vi "Create Group Logger.vi"(7 "Timestamp":string, 8 "error in (no error)":errorcluster, 10 "Group":refnum<class "Group.lvclass">, 11 "Historian Logger in":refnum<class "Historian Logger.lvclass">) -> (0 "error out":errorcluster, 3 "Historian Logger out":refnum<class "Historian Logger.lvclass">)   [LabVIEW 2020, in "VolatusHistorian.lvlib" / "Historian Logger.lvclass"]
uses:
  Historian Logger.lvclass
  C:/dev/lv20CE/relink/lv-volatus/Volatus/Module/Module.lvclass
  lv-vecto/Vecto/Group/Group.lvclass
  Group Buffer DBL/Group Buffer DBL.lvclass
  Volatus/Module/Module.lvclass/Module.ctl
  lv-vecto/Vecto/Group/Group.lvclass/Group.ctl
  lv-vecto/Vecto/Group Config/Group Config.lvclass/Group Config.ctl
  lv-vecto/Vecto/Group DBL/Group DBL.lvclass
  Group Info.ctl
  Volatus/MessageQ/MessageQ.lvclass
  VolatusData/Logger State.ctl
  VolatusConfig/VolatusConfigElement/VolatusConfigElement.lvclass
  Historian Logger.lvclass/Historian Logger.ctl
  VolatusData/Data Logger DBL Module/Data Logger DBL Module.lvclass
  Volatus/Module/Module.lvclass
  VolatusData/VolatusData.lvlib
  C:/dev/lv20CE/relink/lv-volatus/VolatusHistorian/Historian Logger/Historian Logger.lvclass
  C:/dev/lv20CE/relink/lv-volatus/VolatusData/Data Logger DBL Module/Data Logger DBL Module.lvclass
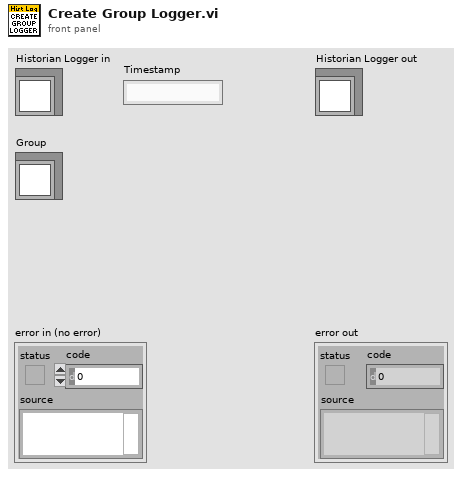
[diagram p1: front panel]
types:
  T1 = typedef "VectoConfig.lvlib/Group Data Type.ctl" = enum16{"Double", "String", "Bool"}
  T2 = typedef "VolatusData.lvlib/Prepare Log.ctl" = cluster{"Folder":path, "Series":string}
  T3 = typedef "VolatusHistorian.lvlib/Historian Logger.lvclass/Group Info.ctl" = cluster{"Buffer":refnum<class "Group Buffer DBL.lvclass">, "Logger":refnum<class "MessageQ.lvclass">, "Group":refnum<class "Group.lvclass">, "Last Timestamp":dbl, "State":T4}
  T4 = typedef "VolatusData.lvlib/Logger State.ctl" = enum16{"Unknown", "Idle", "Preparing", "Ready", "Logging", "Stopping"}
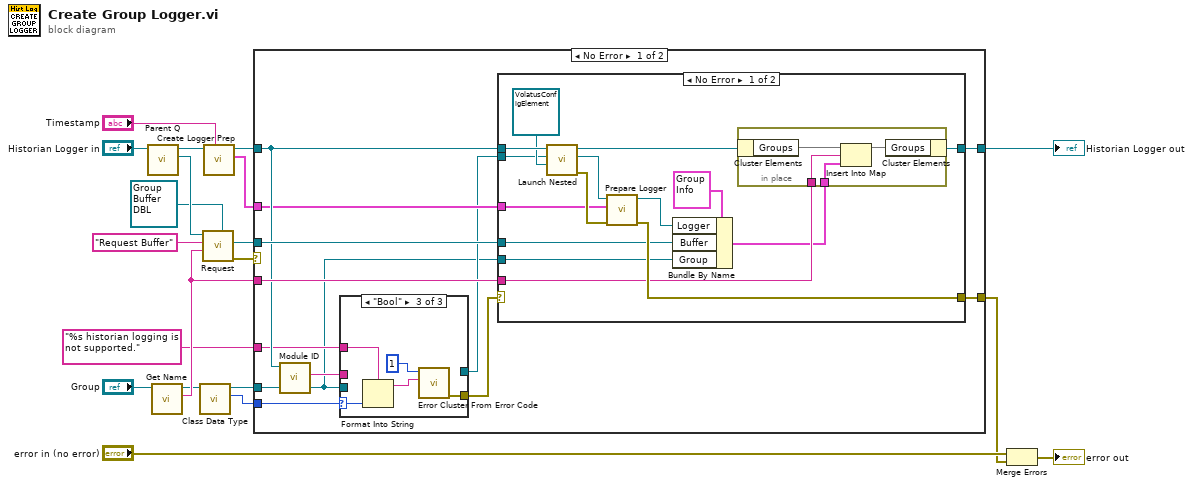
[diagram p0: block diagram]
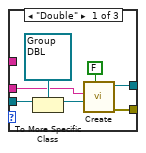
[diagram p2: hidden frame]
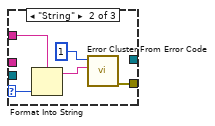
[diagram p3: hidden frame]
diagram:
  n1 = call "Parent Q.vi"("Module in"="Historian Logger in") -> ("Parent Q"=w16:refnum<class "MessageQ.lvclass">, "Module out"=w8:refnum<class "Historian Logger.lvclass">)  [unwired: 9 in]
  n2 = call "Get Name.vi"("Group in"="Group") -> ("Name"=w12:string, "Group out"=w5:refnum<class "Group.lvclass">)  [unwired: 8 in, 1 out]
  n3 = call "Class Data Type.vi"("Group in"=w5) -> ("Class Data Type"=w4:T1, "Group out"=w3:refnum<class "Group.lvclass">)  [unwired: 8 in, 1 out]
  n4 = call "Request.vi"("Response Type (None)"=refnum<class "Group Buffer DBL.lvclass"> refnum ("VolatusHistorian.lvlib:Group Buffer DBL.lvclass"), "Data"=w12, "ID"="Request Buffer", "MessageQ in"=w16) -> ("error out"=w14:errorcluster, "Response"=w13:refnum<class "Group Buffer DBL.lvclass">)  [unwired: 5 in, 1 out]
  n5 = call "Create Logger Prep.vi"("Timestamp"="Timestamp", "Historian Logger in"=w8) -> ("Logger Info"=w6:T2, "Historian Logger out"=w7:refnum<class "Historian Logger.lvclass">)  [unwired: 7 in, 1 out]
  n6 = case shown="No Error" w14 {
    selector: w14 -> [_ w72]
    tunnel: w13 -> [w29 _]
    tunnel: w7 -> [w28 w71]
    tunnel: w12 -> [w30 _]
    tunnel: [w27 w71] -> w11
    tunnel: [w31 w72] -> w9
    tunnel: w6 -> [w26 _]
    tunnel: w4 -> [w25 _]
    tunnel: w3 -> [w21 _]
    tunnel: "%s historian logging is not supported." -> [w23 _]
    frame No Error {
      n7 = call-dynamic "Module ID.vi"("Historian Logger in"=w28) -> ("Module ID"=w24:string)  [unwired: 10 in]
      n8 = case shown="\"Bool\"" w25 {
        selector: w25 -> [_ w42 w47]
        tunnel: w21 -> [w39 _ _]
        tunnel: w24 -> [w36 _ _]
        tunnel: [w34 w44 w49] -> w32
        tunnel: [w33 _ _] -> w22
        tunnel: w23 -> [_ w41 w46]
        frame "Double" {
          n9 = To More Specific Class(target class=refnum<class "Group DBL.lvclass"> refnum ("Group"), reference=w39) -> (specific class reference=w38:refnum<class "Group DBL.lvclass">)  [unwired: 1 in, 1 out]
          n10 = call "Create.vi"("Use Manager (T)"=FALSE, "Group"=w38, "Parent Name"=w36) -> ("error out"=w34:errorcluster, "Data Logger Module out"=w33:refnum<class "Data Logger DBL Module.lvclass">)  [unwired: 7 in]
        }
        frame "String" {
          n11 = Format Into String(format string=w41, w42) -> (resulting string=w40:string)  [unwired: 2 in, 1 out]
          n12 = call <vilib>:"Error Cluster From Error Code.vi"("error message (\"\")"=w40, "error code (0)"=1) -> ("error out"=w44:errorcluster)  [unwired: 7 in]
        }
        frame "Bool" {
          n13 = Format Into String(format string=w46, w47) -> (resulting string=w45:string)  [unwired: 2 in, 1 out]
          n14 = call <vilib>:"Error Cluster From Error Code.vi"("error message (\"\")"=w45, "error code (0)"=1) -> ("error out"=w49:errorcluster)  [unwired: 7 in]
        }
      }
      n15 = case shown="No Error" w32 {
        selector: w32 -> [_ w69]
        tunnel: [w64 w69] -> w31
        tunnel: w30 -> [w62 _]
        tunnel: w29 -> [w60 _]
        tunnel: w28 -> [w59 w70]
        tunnel: [w56 w70] -> w27
        tunnel: w26 -> [w53 _]
        tunnel: w22 -> [w51 _]
        tunnel: w21 -> [w50 _]
        frame No Error {
          n16 = call "Launch Nested.vi"("Config Element"=refnum<class "VolatusConfigElement.lvclass"> refnum, "Nested Module"=w51, "Parent in"=w59) -> ("error out"=w63:errorcluster, "MessageQ"=w54:refnum<class "MessageQ.lvclass">, "Parent out"=w58:refnum<class "Historian Logger.lvclass">)  [unwired: 6 in]
          n17 = call "Prepare Logger.vi"("error in (no error)"=w63, "Prepare Log"=w53, "MsgQ in"=w54) -> ("error out"=w64:errorcluster, "MsgQ"=w52:refnum<class "MessageQ.lvclass">)  [unwired: 7 in]
          n18 = Bundle By Name(cluster=T3 {"Buffer"=refnum, "Logger"=refnum, "Group"=refnum, "Last Timestamp"=0.0, "State"=enum."Unknown"} ("Group Info"), "Logger"=w52, "Buffer"=w60, "Group"=w50) -> (w57:T3)
          n19 = in-place {
            in-place-border: w62 -> [w66]
            in-place-border: w57 -> [w65]
            n20 = in-place-cluster #1(w58) -> ("Groups"=w68:map{string, T3})
            n21 = Insert Into Map(map in=w68, key=w66, value=w65) -> (map out=w67:map{string, T3})  [unwired: 2 out]
            n22 = in-place-cluster #1("Groups"=w67) -> (w56:refnum<class "Historian Logger.lvclass">)
          }
        }
        frame Error {
        }
      }
    }
    frame Error {
    }
  }
  "Historian Logger out" <- w11
  n23 = Merge Errors("error in (no error)", w9) -> (→"error out":errorcluster)
